vi "F.L.Y Stick Controller.vi"   [LabVIEW 2019]
uses:
  <vilib>/Rock Robotics/WPI/Joystick/WPI_JoystickDeviceEnum.ctl
  F.L.Y Stick Controller Global.vi
types:
  T1 = typedef "WPI_JoystickDeviceEnum.ctl" = enum16{"USB 0", "USB 1", "USB 2", "USB 3", "USB 4", "USB 5"}
  T2 = typedef "WPI_JoystickDevRef.ctl" = cluster{"Device":T1}
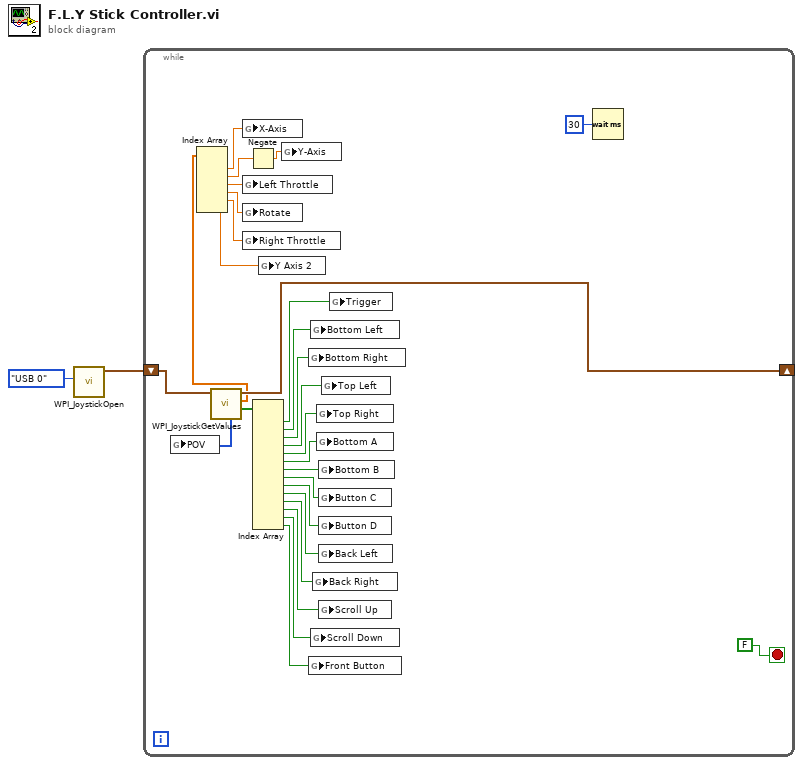
[diagram p0: block diagram]
diagram:
  n1 = call <vilib>:"WPI_JoystickOpen.vi"("JoystickDevice"=WPI_JoystickDeviceEnum."USB 0") -> ("JoystickDevRef"=w2:T2)  [unwired: 10 in]
  n2 = while {
    shift-right: [w28] -> _
    shift-left: w2 -> [w29]
    stop <- FALSE stop-if-true
    n3 = call <vilib>:"WPI_JoystickGetValues.vi"("JoystickDevRef"=w29) -> ("Buttons"=w27:bool[], "Axes"=w12:dbl[], "JoystickDevRef"=w28:T2, "POVs"=w7:i16[])  [unwired: 6 in, 1 out]
    n4 = global write "F.L.Y Stick Controller Global.vi" "POV"(w7) -> ()
    n5 = Index Array(array=w12) -> (element #1=w11:dbl, element #2=w4:dbl, element #3=w10:dbl, element #4=w9:dbl, element #5=w8:dbl, element #6=w3:dbl)  [unwired: 6 in]
    n6 = global write "F.L.Y Stick Controller Global.vi" "X-Axis"(w11) -> ()
    n7 = global write "F.L.Y Stick Controller Global.vi" "Left Throttle"(w10) -> ()
    n8 = global write "F.L.Y Stick Controller Global.vi" "Rotate"(w9) -> ()
    n9 = global write "F.L.Y Stick Controller Global.vi" "Right Throttle"(w8) -> ()
    n10 = Negate(x=w4) -> (-x=w5:dbl)
    n11 = Index Array(array=w27) -> (element #1=w26:bool, element #2=w25:bool, element #3=w24:bool, element #4=w23:bool, element #5=w22:bool, element #6=w21:bool, element #7=w20:bool, element #8=w19:bool, element #9=w18:bool, element #10=w17:bool, element #11=w16:bool, element #12=w15:bool, element #13=w14:bool, element #14=w13:bool)  [unwired: 14 in]
    n12 = global write "F.L.Y Stick Controller Global.vi" "Y Axis 2"(w3) -> ()
    n13 = global write "F.L.Y Stick Controller Global.vi" "Y-Axis"(w5) -> ()
    n14 = global write "F.L.Y Stick Controller Global.vi" "Bottom Right"(w24) -> ()
    n15 = global write "F.L.Y Stick Controller Global.vi" "Front Button"(w13) -> ()
    n16 = global write "F.L.Y Stick Controller Global.vi" "Bottom Left"(w25) -> ()
    n17 = global write "F.L.Y Stick Controller Global.vi" "Scroll Down"(w14) -> ()
    n18 = global write "F.L.Y Stick Controller Global.vi" "Back Right"(w16) -> ()
    n19 = global write "F.L.Y Stick Controller Global.vi" "Top Right"(w22) -> ()
    n20 = global write "F.L.Y Stick Controller Global.vi" "Bottom A"(w21) -> ()
    n21 = global write "F.L.Y Stick Controller Global.vi" "Bottom B"(w20) -> ()
    n22 = global write "F.L.Y Stick Controller Global.vi" "Button C"(w19) -> ()
    n23 = global write "F.L.Y Stick Controller Global.vi" "Button D"(w18) -> ()
    n24 = global write "F.L.Y Stick Controller Global.vi" "Back Left"(w17) -> ()
    n25 = global write "F.L.Y Stick Controller Global.vi" "Scroll Up"(w15) -> ()
    n26 = global write "F.L.Y Stick Controller Global.vi" "Top Left"(w23) -> ()
    n27 = global write "F.L.Y Stick Controller Global.vi" "Trigger"(w26) -> ()
    n28 = Wait (ms)(milliseconds to wait=u32 30) -> ()  [unwired: 1 out]
  }
